vi "example_VL Transmit.vi"() -> ()   [LabVIEW 2020]
uses:
  src/_controls/comm_computedMAC-IP.ctl
  src/_controls/comm_udp_tx.ctl
  src/_controls/comm_config_vl_tx.ctl
  src/helpers/EthFrameManagement/controls/mac_src_info_afdx.ctl
  src/_polimorphicInstances/session/CreateSession(Tx-UDP Port-Oriented).vi
  src/bsp/AFDX_Transmit/Create Tx VL.vi
  src/_polimorphicInstances/udpPort/CreateUdpPort(TX-CommPort).vi
  src/AIM664LV.lvlib
  src/helpers/EthFrameManagement/EthFrameManagement.lvlib
panel:
  in  "VlTx":T1={"domainID"=0, "sideID"=0, "locationID"=0, "interfaceID"=1}
  out "Duplicated":bool
  in  "VL Config":T2[](array[typedef]) {"NetSelect" items=["FDX_TX_FRAME_DLY_A"=0, "FDX_TX_FRAME_DLY_B"=1, "FDX_TX_FRAME_BOTH "=3, "FDX_TX_FRAME_ONLY_A"=4, "FDX_TX_FRAME_ONLY_B "=5]; "interfaceID" format="%.0b"}
  in  "CommPort Config":T3[](array[typedef])
  in  "millisecond multiple":u32=128
  in  "PortMap":u32
  out "size(s)":i32
  out "IndexCycleCount":u32[](array[numeric])
  out "MsgCount":u32[](array[numeric])
  out "CurrentIndex":u32[](array[numeric])
  out "BytesWritten":u32[](array[numeric])
  in  "port":u32
  in  "board":u32
  out "current time":timestamp=timestamp(3677762637.591913 s since 1904-01-01)
  out "current irig time":T4={"SignOut"=40, "DayOut"=1, "HourOut"=1, "MinOut"=28, "SecondOut"=39, "MilliSecOut"=539, "MicroSecOut"=300, "NanoSecOut"=0, "InfoOut"=0, "Mode"=3}
  out "CommPort Addresses":T5[](array[typedef]) {"MACsrc" format="%.0x"}
  in  "Data":u8[](array[numeric])=[255, 255, 255, 255, 255, 255, 255, 255, 255, 255, 255, 255, 255, 255, 255, 255, 255, 255, 255, 255, 255, 255, 255, 255, 255, 255, 255, 255, 255, 255, 255, 255, 255, 255, 255, 255, 255, 255, 255, 255, 255, 255, 255, 255, 255, 255, 255, 255, 255, 255, 255, 255, 255, 255, 255, 255, 255, 255, 255, 255, 255, 255, 255, 255, 255, 255, 255, 255, 255, 255, 255, 255, 255, 255, 255, 255, 255, 255, 255, 255, 255, 255, 255, 255, 255, 255, 255, 255, 255, 255, 255, 255, 255, 255, 255, 255, 255, 255, 255, 170] format="%.0x"
  in  "stop":bool
  out "PortInitOut":T6={"PortConfig"=0, "PortUsed"=1, "GlobalMemFree"=0, "SharedMemFree"=0} {"PortConfig" items=["FDX_SINGLE", "FDX_REDUNDANT"]}
  out "error out":errorcluster
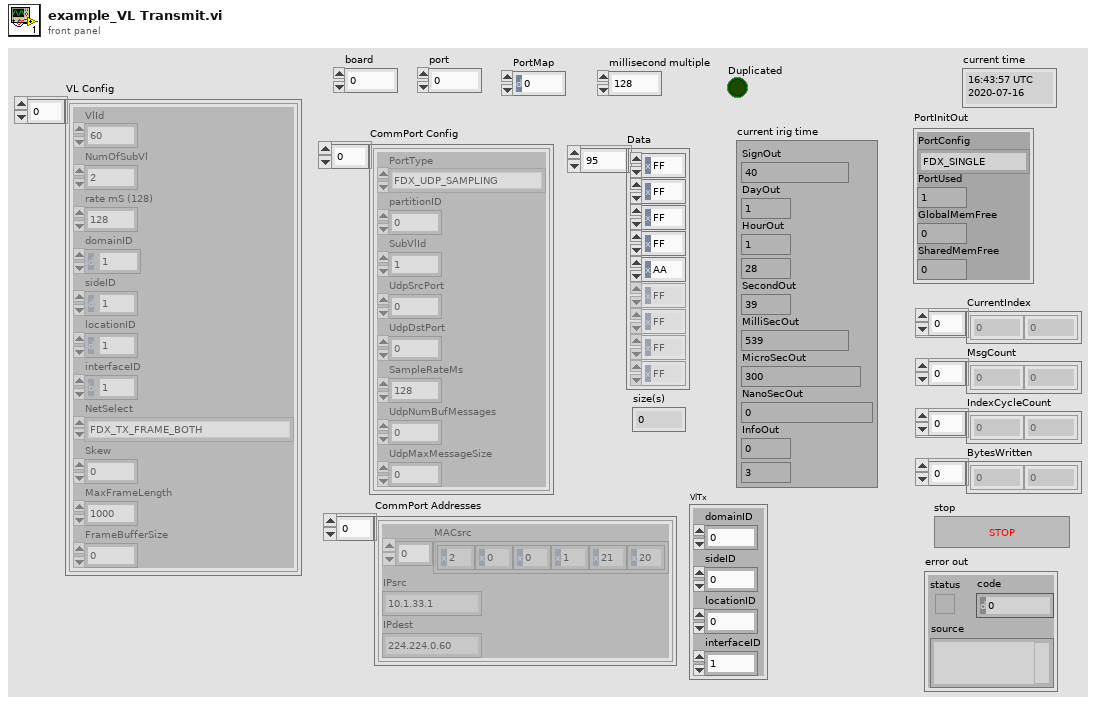
[diagram p1: front panel]
types:
  T1 = typedef "EthFrameManagement.lvlib/mac_src_info_afdx.ctl" = cluster{"domainID":u8, "sideID":u8, "locationID":u8, "interfaceID":u8}
  T2 = typedef "AIM664LV.lvlib/comm_config_vl_tx.ctl" = cluster{"VlId":u16, "NumOfSubVl":u16, "rate mS (128)":dbl, "domainID":u8, "sideID":u8, "locationID":u8, "interfaceID":u8, "NetSelect":u32, "Skew":u32, "MaxFrameLength":u32, "FrameBufferSize":u32}
  T3 = typedef "AIM664LV.lvlib/comm_udp_tx.ctl" = cluster{"PortType":enum16{"FDX_UDP_SAMPLING", "FDX_UDP_QUEUING"}, "partitionID":u8, "SubVlId":u8, "UdpSrcPort":u16, "UdpDstPort":u16, "SampleRateMs":dbl, "UdpNumBufMessages":u32, "UdpMaxMessageSize":u32}
  T4 = cluster{"SignOut":i32, "DayOut":u32, "HourOut":u32, "MinOut":u32, "SecondOut":u32, "MilliSecOut":u32, "MicroSecOut":u32, "NanoSecOut":u32, "InfoOut":u32, "Mode":u32}
  T5 = typedef "AIM664LV.lvlib/comm_computedMAC-IP.ctl" = cluster{"MACsrc":u8[], "IPsrc":string, "IPdest":string}
  T6 = cluster{"PortConfig":u32, "PortUsed":u32, "GlobalMemFree":u32, "SharedMemFree":u32}
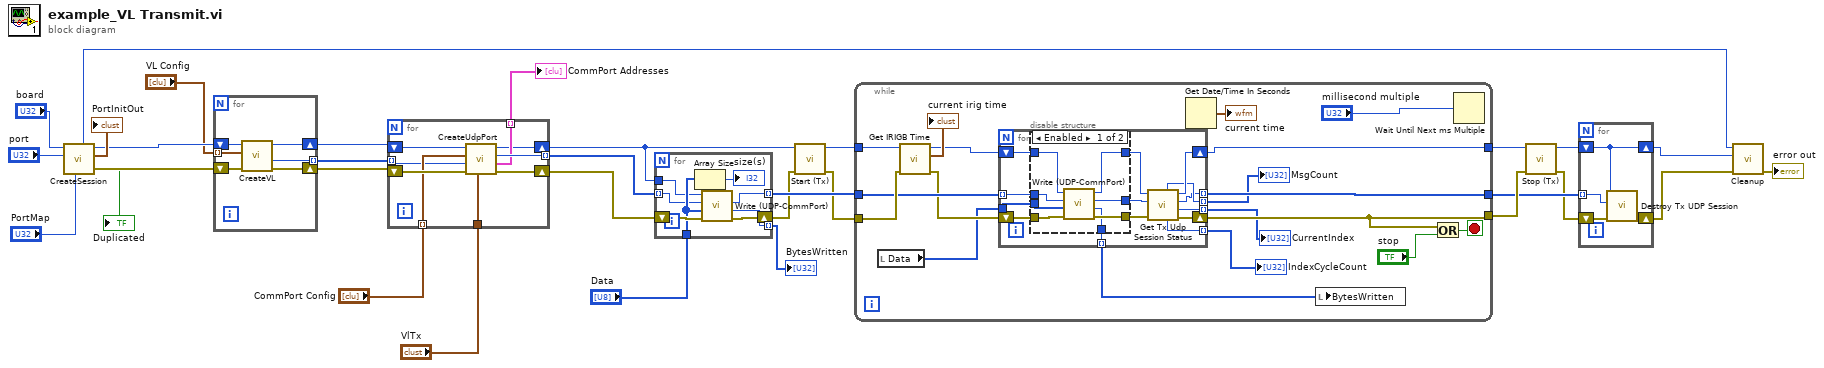
[diagram p0: block diagram]
diagram:
  n1 = call-poly "CreateSession.vi"("PortMap"="PortMap", "port"="port", "board"="board") -> ("error out"=w13:errorcluster, "PortInitOut"=→"PortInitOut":T6, "port handle out"=w14:u32, "Duplicated"=→"Duplicated":bool, "InstrumentHandle_board out"=w2:u32)  [unwired: 4 in]
  n2 = for {
    tunnel: [w34] -> w10 mode=indexing
    tunnel: "VL Config" -> [w33] mode=indexing
    shift-right: [w36] -> w12
    shift-left: w14 -> [w38]
    shift-right: [w35] -> w11
    shift-left: w13 -> [w37]
    n3 = call-poly "CreateVL.vi"("error in (no error)"=w37, "VL Config"=w33, "InstrumentHandle in"=w38) -> ("error out"=w35:errorcluster, "VlId"=w34:u16, "InstrumentHandle out"=w36:u32)  [unwired: 6 in]
  }
  n4 = for {
    tunnel: [w46] -> w30 mode=indexing
    tunnel: [w43] -> w26 mode=indexing
    shift-right: [w42] -> w6
    shift-left: w12 -> [w47]
    shift-right: [w45] -> w28
    shift-left: w11 -> [w44]
    tunnel: w10 -> [w40] mode=indexing
    tunnel: "CommPort Config" -> [w41] mode=indexing
    tunnel: "VlTx" -> [w39]
    n5 = call-poly "CreateUdpPort.vi"("VlTx"=w39, "error in (no error)"=w44, "VlId"=w40, "CommPort Config"=w41, "port handle in"=w47) -> ("error out"=w45:errorcluster, "computedAddresses"=w43:T5, "commPort handle out"=w46:u32, "port handle out"=w42:u32)  [unwired: 3 in]
  }
  "CommPort Addresses" <- w26
  n6 = for {
    tunnel: "Data" -> [w51]
    tunnel: [w53] -> w16 mode=indexing
    shift-right: [w54] -> w24
    shift-left: w28 -> [w55]
    tunnel: w30 -> [w50] mode=indexing
    tunnel: [w48] -> w29 mode=indexing
    tunnel: w6 -> [w49]
    n7 = Array Size(array=w51) -> (size(s)=→"size(s)":i32)
    n8 = call "Write (UDP-CommPort).vi"("error in (no error)"=w55, "Data"=w51, "UdpHandle in"=w50, "InstrumentHandle_port in"=w49) -> ("error out"=w54:errorcluster, "BytesWritten"=w53:u32, "UdpHandle out"=w48:u32)  [unwired: 4 in, 1 out]
  }
  "BytesWritten" <- w16
  n9 = call "Start (Tx).vi"("error in (no error)"=w24, "InstrumentHandle_port in"=w6) -> ("error out"=w23:errorcluster, "InstrumentHandle_port out"=w22:u32)  [unwired: 8 in]
  n10 = while {
    tunnel: w23 -> [w69]
    tunnel: w29 -> [w61]
    tunnel: w22 -> [w70]
    tunnel: [w56] -> w25
    tunnel: [w66] -> w19
    tunnel: [w65] -> w20
    stop <- w72 stop-if-true
    n11 = local read "Data"() -> (w58:u8[])
    n12 = call "Get IRIGB Time.vi"("error in (no error)"=w69, "InstrumentHandle_board in"=w70) -> ("error out"=w60:errorcluster, "Curent Irig Time"=→"current irig time":T4, "InstrumentHandle_board out"=w57:u32)  [unwired: 7 in]
    n13 = for {
      tunnel: [w76] -> w66 mode=indexing
      tunnel: [w75] -> w64 mode=indexing
      tunnel: [w77] -> w63 mode=indexing
      tunnel: [w74] -> w62 mode=indexing
      tunnel: w61 -> [w86] mode=indexing
      tunnel: [w81] -> w59 mode=indexing
      tunnel: w58 -> [w83]
      shift-right: [w87] -> w65
      shift-left: w60 -> [w85]
      shift-right: [w78] -> w56
      shift-left: w57 -> [w82]
      n14 = disable-structure shown="Enabled" {
        disable-tunnel: w86 -> [w92 w97]
        disable-tunnel: w85 -> [w95 w96]
        disable-tunnel: [w94 w96] -> w84
        disable-tunnel: [w88 w97] -> w80
        disable-tunnel: w83 -> [w93 _]
        disable-tunnel: w82 -> [w91 _]
        disable-tunnel: [w90 _] -> w81
        disable-tunnel: [w89 _] -> w79
        frame Enabled {
          n15 = call "Write (UDP-CommPort).vi"("error in (no error)"=w95, "Data"=w93, "UdpHandle in"=w92, "InstrumentHandle_port in"=w91) -> ("error out"=w94:errorcluster, "BytesWritten"=w90:u32, "UdpHandle out"=w88:u32, "InstrumentHandle_port out"=w89:u32)  [unwired: 4 in]
        }
        frame Disabled {
        }
      }
      n16 = call "Get Tx Udp Session Status.vi"("error in (no error)"=w84, "UdpHandle in"=w80, "InstrumentHandle_port in"=w79) -> ("error out"=w87:errorcluster, "CurrentIndex"=w75:u32, "UdpHandle out"=w76:u32, "InstrumentHandle_port out"=w78:u32, "IndexCycleCount"=w74:u32, "MsgCount"=w77:u32)  [unwired: 3 in]
    }
    "CurrentIndex" <- w64
    "MsgCount" <- w63
    "IndexCycleCount" <- w62
    n17 = Get Date/Time In Seconds() -> (seconds since 1Jan1904=→"current time":timestamp)
    n18 = local write "BytesWritten"(w59) -> ()
    n19 = Or(x=w65, y="stop") -> (x .or. y?=w72:bool)
    n20 = Wait Until Next ms Multiple(millisecond multiple="millisecond multiple") -> ()  [unwired: 1 out]
  }
  n21 = call "Stop (Tx).vi"("error in (no error)"=w20, "InstrumentHandle_port in"=w25) -> ("error out"=w18:errorcluster, "InstrumentHandle_port out"=w5:u32)  [unwired: 8 in]
  n22 = for {
    tunnel: w19 -> [w99] mode=indexing
    shift-right: [w100] -> w17
    shift-left: w18 -> [w101]
    shift-right: [w98] -> w4
    shift-left: w5 -> [w98]
    n23 = call "Destroy Tx UDP Session.vi"("error in (no error)"=w101, "UdpHandle in"=w99, "InstrumentHandle_port in"=w98) -> ("error out"=w100:errorcluster)  [unwired: 7 in, 1 out]
  }
  n24 = call "Cleanup.vi"("error in (no error)"=w17, "InstrumentHandle_port in"=w4, "InstrumentHandle_board in"=w2) -> ("error out"=→"error out":errorcluster)  [unwired: 8 in]
